vi "Write Working Directory.vi"(8 "error in (no error)":errorcluster, 10 "Working Directory":path, 11 "Console Wrapper in":refnum<class "Console Wrapper.lvclass">) -> (0 "error out":errorcluster, 3 "Console Wrapper out":refnum<class "Console Wrapper.lvclass">)   [LabVIEW 2020, in "Console Wrapper.lvclass"]
uses:
  Console Wrapper.lvclass
  Console Wrapper.lvclass/Console Wrapper.ctl
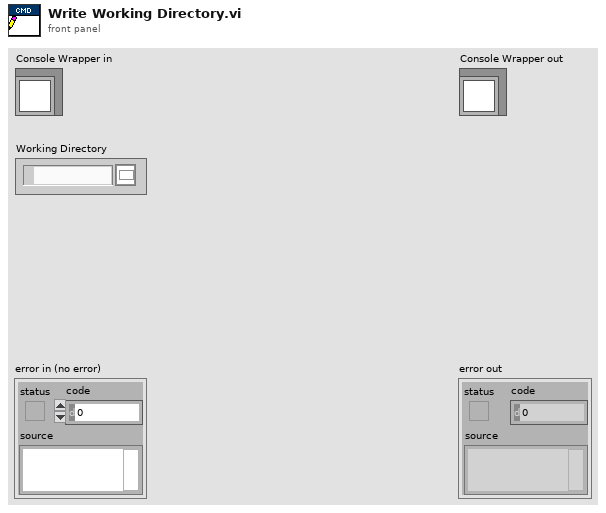
[diagram p1: front panel]
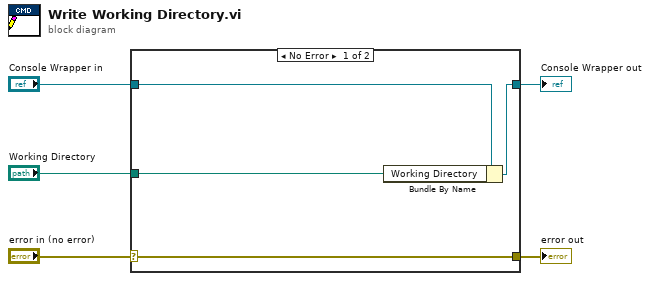
[diagram p0: block diagram]
diagram:
  n1 = case shown="No Error" "error in (no error)" {
    selector: "error in (no error)" -> [w9 w10]
    tunnel: [w9 w10] -> w4
    tunnel: [w7 w11] -> w2
    tunnel: "Console Wrapper in" -> [w8 w11]
    tunnel: "Working Directory" -> [w6 _]
    frame No Error {
      n2 = Bundle By Name(cluster=w8, "Working Directory"=w6) -> (w7:refnum<class "Console Wrapper.lvclass">)
    }
    frame Error {
    }
  }
  "error out" <- w4
  "Console Wrapper out" <- w2
